vi "Write Binary Config.vi"(4 "Include Class Name":bool, 6 "byte order (0:big-endian, network order)":T1(ring), 8 "error in (no error)":errorcluster, 11 "Concatenate_STR in":refnum<class "Concatenate_STR.lvclass">) -> (0 "error out":errorcluster, 2 "Binary":string, 3 "Concatenate_STR out":refnum<class "Concatenate_STR.lvclass">)   [LabVIEW 2021, in "Concatenate_STR.lvclass"]
uses:
  Concatenate_STR.lvclass
  Concatenate_STR.lvclass/Concatenate_STR.ctl
  Abs_Types/String/Abs_String.lvclass
  Abs_Types/Value/Abs_Value.lvclass
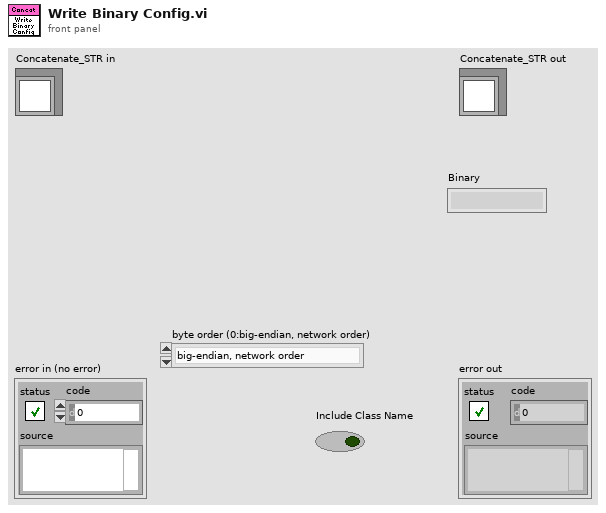
[diagram p1: front panel]
types:
  T1 = enum16{"big-endian, network order", "native, host order", "little-endian"}
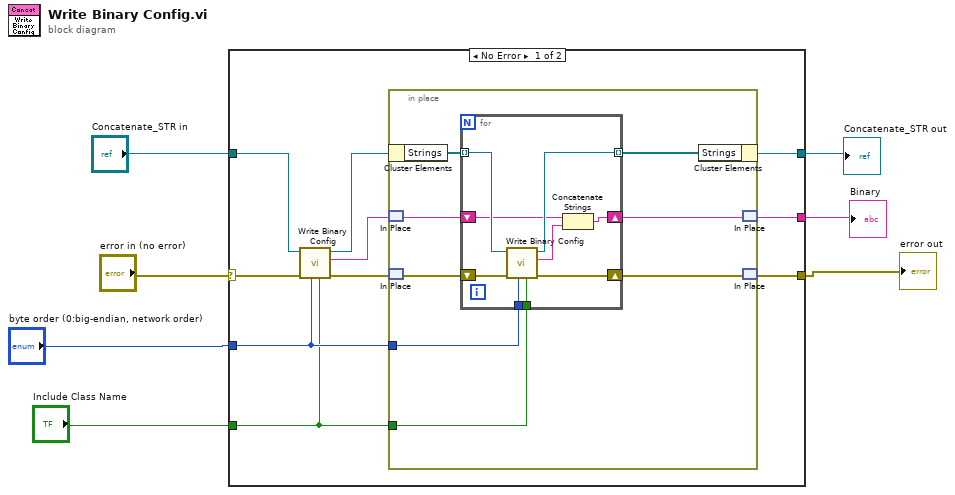
[diagram p0: block diagram]
diagram:
  n1 = case shown="No Error" "error in (no error)" {
    selector: "error in (no error)" -> [w17 w35]
    tunnel: "Concatenate_STR in" -> [w16 w36]
    tunnel: [w12 _] -> w3
    tunnel: "byte order (0:big-endian, network order)" -> [w11 _]
    tunnel: "Include Class Name" -> [w10 _]
    tunnel: [w9 w35] -> w2
    tunnel: [w8 w36] -> w1
    frame No Error {
      n2 = call-parent "Write Binary Config.vi"("Include Class Name"=w10, "byte order (0:big-endian, network order)"=w11, "error in (no error)"=w17, "Abs_Type in"=w16) -> ("error out"=w14:errorcluster, "Binary"=w13:string, "Abs_Type out"=w15:refnum<class "Concatenate_STR.lvclass">)  [unwired: 5 in]
      n3 = in-place {
        in-place-border: w11 -> [w20]
        in-place-border: w10 -> [w22]
        n4 = in-place-cluster #1(w15) -> ("Strings"=w23:refnum<class "Abs_Value.lvclass">[])
        n5 = in-place-match #2(w13) -> (w18:string)
        n6 = in-place-match #3(w14) -> (w25:errorcluster)
        n7 = for {
          tunnel: [w33] -> w24 mode=indexing
          tunnel: w23 -> [w32] mode=indexing
          tunnel: w22 -> [w31]
          tunnel: w20 -> [w29]
          shift-right: [w30] -> w21
          shift-left: w25 -> [w34]
          shift-right: [w27] -> w19
          shift-left: w18 -> [w26]
          n8 = call-dynamic "Write Binary Config.vi"("Include Class Name"=w31, "byte order (0:big-endian, network order)"=w29, "error in (no error)"=w34, "Abs_Type in"=w32) -> ("error out"=w30:errorcluster, "Binary"=w28:string, "Abs_Type out"=w33:refnum<class "Abs_Value.lvclass">)  [unwired: 5 in]
          n9 = Concatenate Strings(w26, w28) -> (w27:string)
        }
        n10 = in-place-cluster #1("Strings"=w24) -> (w8:refnum<class "Concatenate_STR.lvclass">)
        n11 = in-place-match #2(w19) -> (w12:string)
        n12 = in-place-match #3(w21) -> (w9:errorcluster)
      }
    }
    frame Error {
    }
  }
  "error out" <- w2
  "Concatenate_STR out" <- w1
  "Binary" <- w3
